vi "IRISS_FPGA_IO_RIO.vi"() -> ()   [LabVIEW 2016]
doc: "This VI contains a basic quadrature decoder which is reset asynchronously upon clicking the reset button."
uses:
  <vilib>/Platform/TimedLoop/XDataNode/timing_clust.ctl
  <vilib>/Platform/TimedLoop/XDataNode/nitl_modes.ctl
  <vilib>/Platform/TimedLoop/XDataNode/wakeup.ctl
  <vilib>/rvi/Emulation/niFpgaGetClockAttributes.vi
  <vilib>/rvi/Emulation/niFpgaSctlEmulationGetInTimedLoop.vi
  <vilib>/rvi/Emulation/niFpgaEmulationReportErrorSimple.vi
  <vilib>/rvi/eio/common/nirviEmuTemplateMethod_errors.vi
  <vilib>/rvi/Emulation/niFpgaCriticalErrorInLSC.vi
  <vilib>/eio/EIONode/EIONode.xnode
  <vilib>/platform/TimedLoop/XDataNode/XDataNode.xnode
  <vilib>/Platform/TimedLoop/XDataNode/XDNodeRunTimeDep.lvlib
  Library/KevinLibraryAll/labview/KevLib01.lvlib
panel:
  in  "Reset 9":bool
  in  "Reset 10":bool
  in  "Reset 14":bool
  in  "Period (Ticks)":u32=2000
  out "Home OCT z":bool
  in  "DIR Y":bool
  in  "INHB Y":bool
  out "FAULT Y":bool
  out "Position Y":i32
  out "JumpBy2Error Y":i16
  in  "Reset Y":bool
  in  "Y DC":fxp<+,32,0>
  in  "DIR X":bool
  in  "INHB X":bool
  out "FAULT X":bool
  out "Position X":i32
  out "JumpBy2Error X":i16
  in  "Reset X":bool
  in  "DIR Z":bool
  in  "INHB Z":bool
  out "FAULT Z":bool
  out "Position Z":i32
  out "JumpBy2Error Z":i16
  in  "Reset Z":bool
  in  "Z DC":fxp<+,32,0>
  in  "X DC":fxp<+,32,0>
  out "Home L4":bool
  out "Home L1":bool
  out "Home L2":bool
  out "Home L3":bool
  in  "Positive Direction C1-4":bool
  out "JumpBy2Error C1-4":i16
  out "32 bit Position C1-4":i32
  in  "Reset C1-4":bool
  in  "Positive Direction C1-1":bool
  out "JumpBy2Error C1-1":i16
  out "32 bit Position C1-1":i32
  in  "Reset C1-1":bool
  out "32 bit Position 17":i32
  in  "Reset 17":bool
  in  "Positive Direction 17":bool
  out "JumpBy2Error 17":i16
  out "32 bit Position 16":i32
  in  "Reset 16":bool
  in  "Positive Direction 16":bool
  out "JumpBy2Error 16":i16
  out "32 bit Position 15":i32
  in  "Reset 15":bool
  in  "Positive Direction 15":bool
  out "JumpBy2Error 15":i16
  out "32 bit Position 13":i32
  in  "Reset 13":bool
  in  "Positive Direction 13":bool
  out "JumpBy2Error 13":i16
  in  "Reset 12":bool
  in  "Reset 11":bool
  out "JumpBy2Error 3":i16
  in  "Positive Direction 3":bool
  out "JumpBy2Error 1":i16
  in  "Positive Direction 1":bool
  out "AI":i16[](array[numeric])
  out "32 bit Position 3":i32
  in  "Reset 3":bool
  in  "AO":i16[](array[numeric])=[0, 0, 0, 0, 0, 0, 0, 0]
  out "32 bit Position 1":i32
  in  "Reset 1":bool
  # "Accurus Buttons"
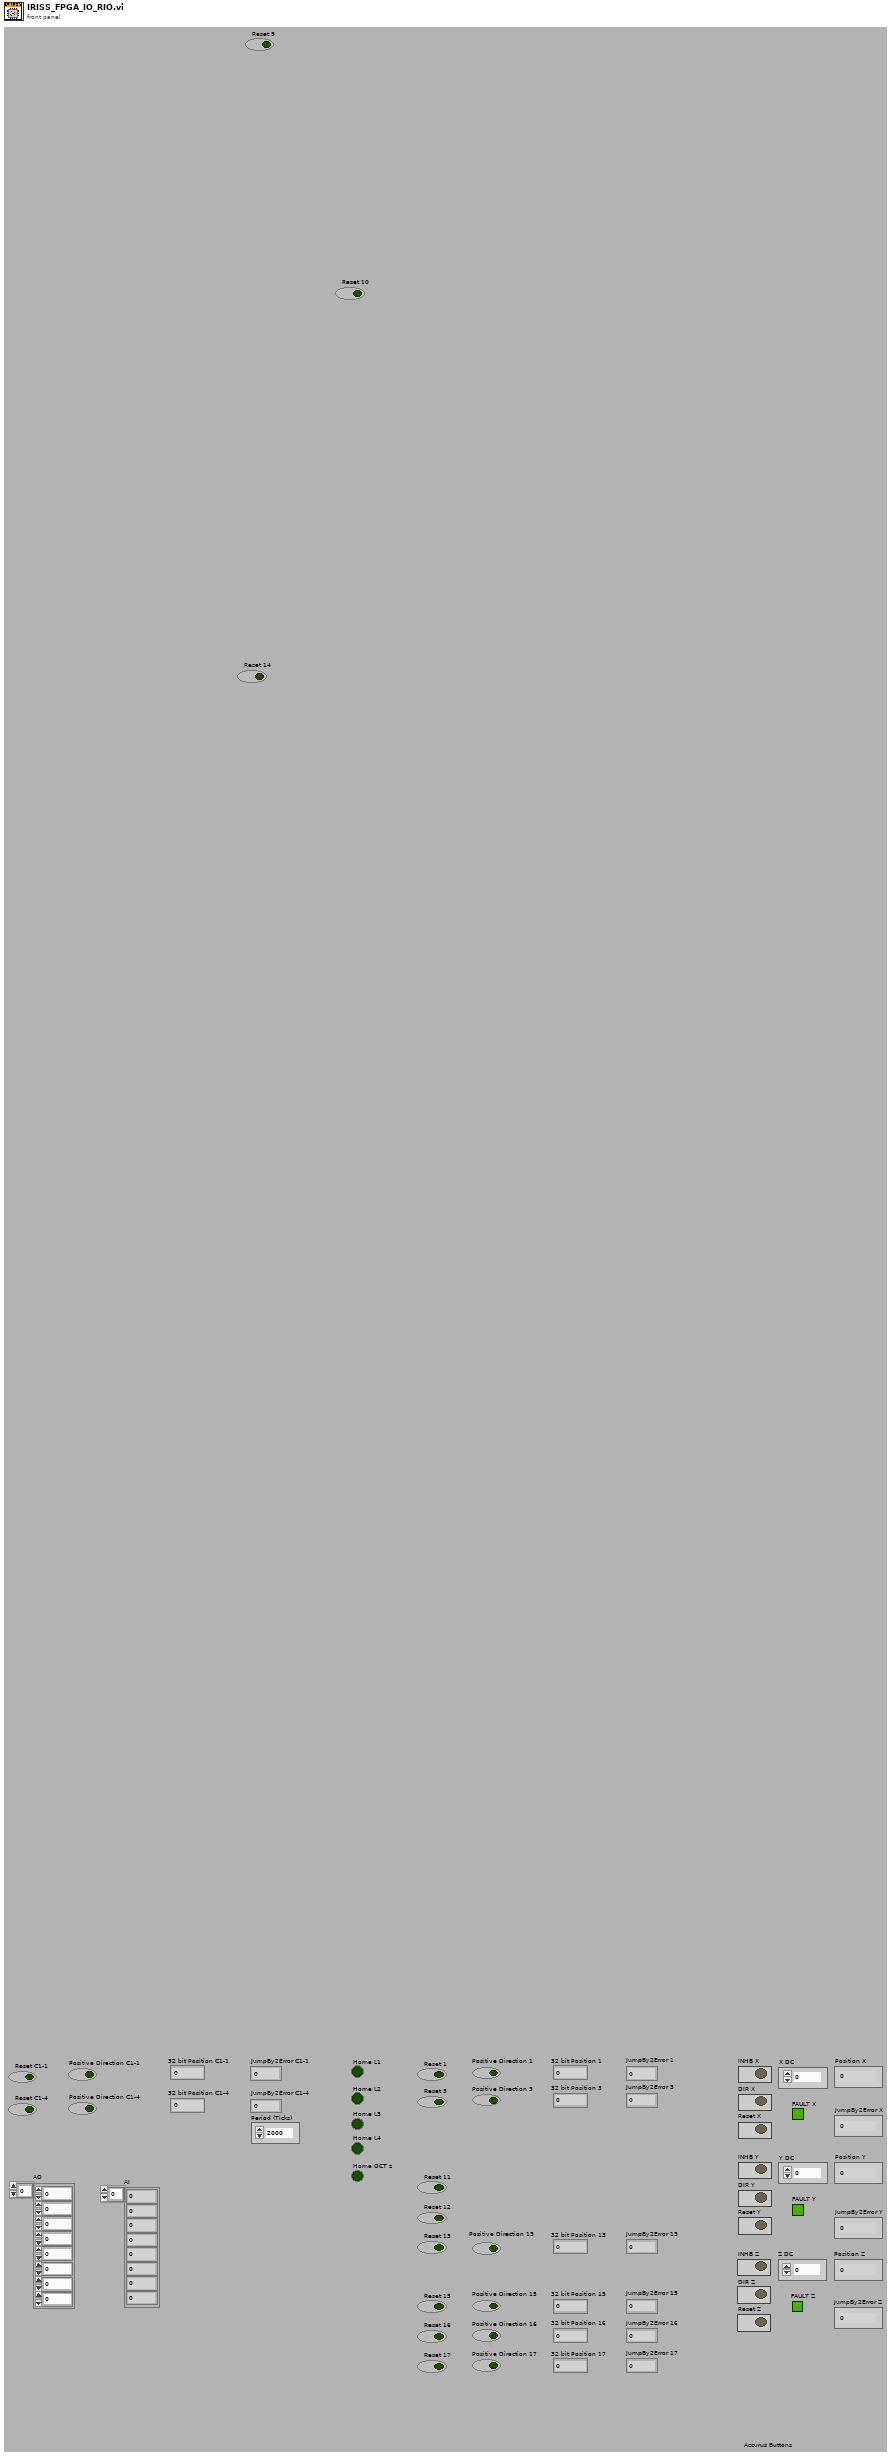
[diagram p1: front panel]
types:
  T1 = typedef "XDNodeRunTimeDep.lvlib/timing_clust.ctl" = cluster{"Expected End [f-1]":u64, "Actual End [f-1]":u64, "Finished Late? [f-1]":bool, "Expected End [i-1]":u64, "Actual End [i-1]":u64, "Finished Late? [i-1]":bool, "Expected Start [i]":u64, "Actual Start [i]":u64, "Expected Start [f]":u64, "Actual Start [f]":u64, "Source Name":string, "Structure Name":string, "Period":i64, "Deadline":i64, "Offset":i64, "Start":i64, "Priority":i32, "Timeout":i32, "Mode":T2, "Wakeup Reason":T3, "Error":errorcluster, "Source Type":string, "Secondary Source Type":string, "Global End Time":u64, "Global Start Time":u64, "Frame Duration":u64, "Iteration Duration":u64, "Assigned CPU":i32, "I/O Scan Engine Mode":u32}
  T2 = typedef "XDNodeRunTimeDep.lvlib/nitl_modes.ctl" = enum32{"No Change", "Process missed periods, maintain original phase", "Discard missed periods, maintain original phase", "Process missed periods, ignore original phase", "Discard missed periods, ignore original phase"}
  T3 = typedef "XDNodeRunTimeDep.lvlib/wakeup.ctl" = enum32{"Normal", "Aborted", "Asynchronous wakeup", "Timing source error", "Timed loop error", "Timeout"}
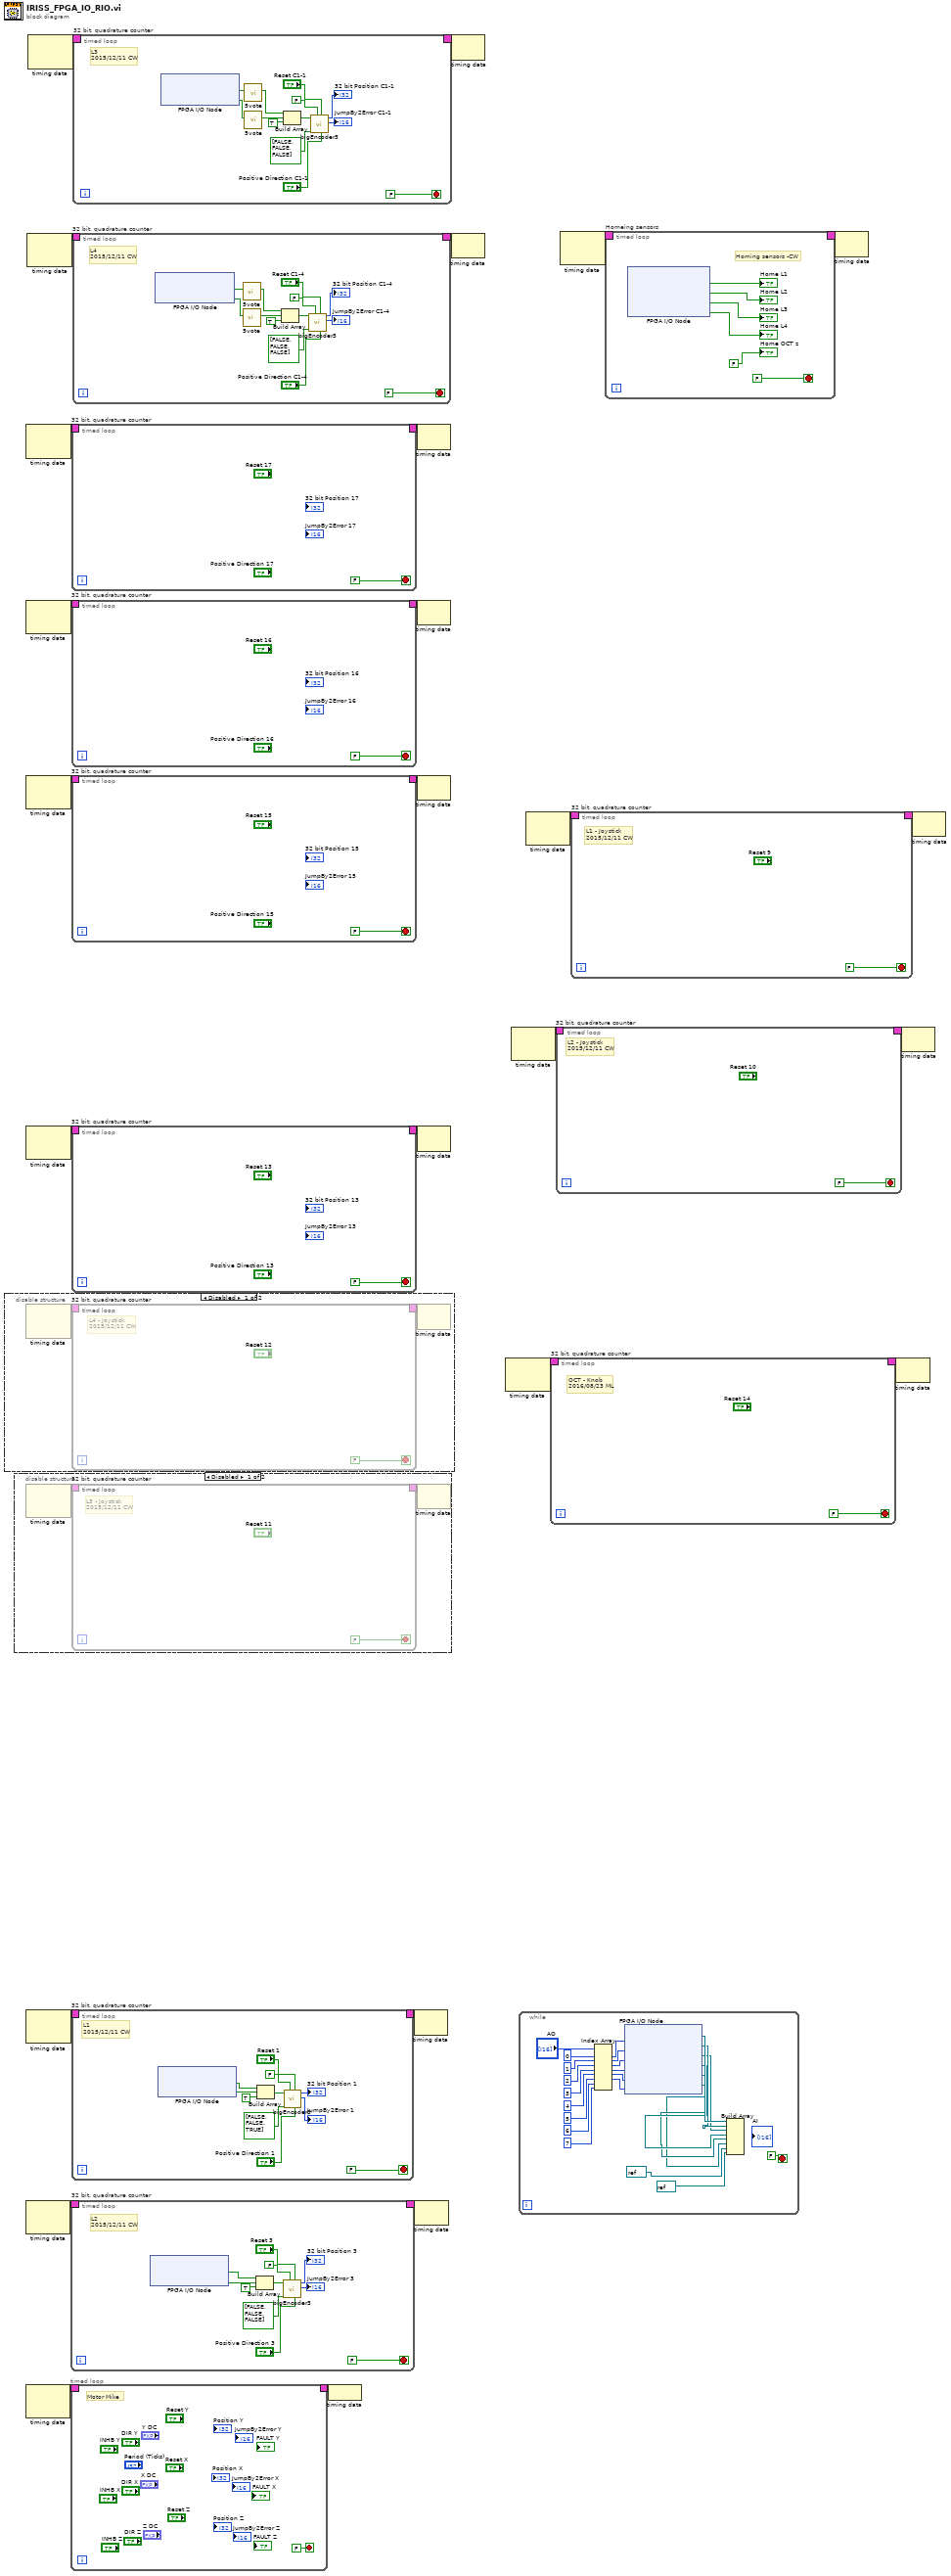
[diagram p0: block diagram]
diagram:
  n1 = disable-structure shown="Disabled" {
    frame Disabled {
      n2 = node-c288() -> (w28:T1)  [unwired: 2 out]
      n3 = timed-loop "32 bit, quadrature counter" {
        timing-out: [_] -> w27
        timing: w28 -> [_]
        stop <- FALSE stop-if-true
        # "L4 - Joystick\n2015/12/11 CW"
      }
      n4 = node-c288(w27) -> ()  [unwired: 1 out]
    }
    frame Enabled {
    }
  }
  n5 = disable-structure shown="Disabled" {
    frame Disabled {
      n6 = node-c288() -> (w35:T1)  [unwired: 2 out]
      n7 = timed-loop "32 bit, quadrature counter" {
        timing-out: [_] -> w34
        timing: w35 -> [_]
        stop <- FALSE stop-if-true
        # "L3 - Joystick\n2015/12/11 CW"
      }
      n8 = node-c288(w34) -> ()  [unwired: 1 out]
    }
    frame Enabled {
    }
  }
  n9 = node-c288() -> (w24:T1)  [unwired: 2 out]
  n10 = node-c288() -> (w8:T1)  [unwired: 2 in]
  n11 = node-c288() -> (w16:T1)  [unwired: 2 out]
  n12 = node-c288() -> (w18:T1)  [unwired: 2 out]
  n13 = node-c288() -> (w20:T1)  [unwired: 2 out]
  n14 = node-c288() -> (w22:T1)  [unwired: 2 out]
  n15 = node-c288() -> (w25:T1)  [unwired: 2 out]
  n16 = node-c288() -> (w12:T1)  [unwired: 2 out]
  n17 = node-c288() -> (w14:T1)  [unwired: 2 out]
  n18 = timed-loop "32 bit, quadrature counter" {
    timing-out: [_] -> w23
    timing: w24 -> [_]
    stop <- FALSE stop-if-true
    # "L2\n2015/12/11 CW"
    n19 = xnode "FPGA I/O Node"() -> ("ConnectorA/DIO2"=w44:bool, "ConnectorA/DIO3"=w43:bool)  [unwired: 2 in, 2 out]
    n20 = Build Array(w44, w43, TRUE ("element")) -> (w50:bool[])
    n21 = call "bigEncoder3.vi"("Positive Direction"="Positive Direction 3", "ForceReset"="Reset 3", "Allow C Reset?"=FALSE, "Reset Array"=bool[] [FALSE, FALSE, FALSE], "Encoder Array"=w50) -> ("JumpBy2Error"=→"JumpBy2Error 3":i16, "Position"=→"32 bit Position 3":i32)  [unwired: 5 out]
  }
  n22 = timed-loop {
    timing: w8 -> [_]
    timing-out: [_] -> w7
    stop <- FALSE stop-if-true
    # "Motor Mike"
  }
  n23 = timed-loop "32 bit, quadrature counter" {
    timing-out: [_] -> w15
    timing: w16 -> [_]
    stop <- FALSE stop-if-true
  }
  n24 = timed-loop "32 bit, quadrature counter" {
    timing-out: [_] -> w17
    timing: w18 -> [_]
    stop <- FALSE stop-if-true
  }
  n25 = timed-loop "32 bit, quadrature counter" {
    timing-out: [_] -> w19
    timing: w20 -> [_]
    stop <- FALSE stop-if-true
  }
  n26 = timed-loop "32 bit, quadrature counter" {
    timing-out: [_] -> w21
    timing: w22 -> [_]
    stop <- FALSE stop-if-true
  }
  n27 = timed-loop "32 bit, quadrature counter" {
    timing-out: [_] -> w26
    timing: w25 -> [_]
    stop <- FALSE stop-if-true
    # "L1\n2015/12/11 CW"
    n28 = xnode "FPGA I/O Node"() -> ("ConnectorA/DIO0"=w78:bool, "ConnectorA/DIO1"=w77:bool)  [unwired: 2 in, 2 out]
    n29 = Build Array(w78, w77, TRUE ("element")) -> (w76:bool[])
    n30 = call "bigEncoder3.vi"("Positive Direction"="Positive Direction 1", "ForceReset"="Reset 1", "Allow C Reset?"=FALSE, "Reset Array"=bool[] [FALSE, FALSE, TRUE], "Encoder Array"=w76) -> ("JumpBy2Error"=→"JumpBy2Error 1":i16, "Position"=→"32 bit Position 1":i32)  [unwired: 5 out]
  }
  n31 = timed-loop "32 bit, quadrature counter" {
    timing-out: [_] -> w11
    timing: w12 -> [_]
    stop <- FALSE stop-if-true
    # "L4\n2015/12/11 CW"
    n32 = xnode "FPGA I/O Node"() -> ("ConnectorA/DIO6"=w85:bool, "ConnectorA/DIO7"=w84:bool)  [unwired: 2 in, 2 out]
    n33 = call "5vote.vi"("Input"=w85) -> ("vote5"=w82:bool)  [unwired: 10 in]
    n34 = call "5vote.vi"("Input"=w84) -> ("vote5"=w83:bool)  [unwired: 10 in]
    n35 = Build Array(w82, w83, TRUE ("element")) -> (w93:bool[])
    n36 = call "bigEncoder3.vi"("Positive Direction"="Positive Direction C1-4", "ForceReset"="Reset C1-4", "Allow C Reset?"=FALSE, "Reset Array"=bool[] [FALSE, FALSE, FALSE], "Encoder Array"=w93) -> ("JumpBy2Error"=→"JumpBy2Error C1-4":i16, "Position"=→"32 bit Position C1-4":i32)  [unwired: 5 out]
  }
  n37 = timed-loop "32 bit, quadrature counter" {
    timing-out: [_] -> w13
    timing: w14 -> [_]
    stop <- FALSE stop-if-true
    # "L3\n2015/12/11 CW"
    n38 = xnode "FPGA I/O Node"() -> ("ConnectorA/DIO4"=w100:bool, "ConnectorA/DIO5"=w99:bool)  [unwired: 2 in, 2 out]
    n39 = call "5vote.vi"("Input"=w100) -> ("vote5"=w97:bool)  [unwired: 10 in]
    n40 = call "5vote.vi"("Input"=w99) -> ("vote5"=w98:bool)  [unwired: 10 in]
    n41 = Build Array(w97, w98, TRUE ("element")) -> (w108:bool[])
    n42 = call "bigEncoder3.vi"("Positive Direction"="Positive Direction C1-1", "ForceReset"="Reset C1-1", "Allow C Reset?"=FALSE, "Reset Array"=bool[] [FALSE, FALSE, FALSE], "Encoder Array"=w108) -> ("JumpBy2Error"=→"JumpBy2Error C1-1":i16, "Position"=→"32 bit Position C1-1":i32)  [unwired: 5 out]
  }
  n43 = node-c288(w7) -> ()
  n44 = node-c288(w26) -> ()  [unwired: 1 out]
  n45 = node-c288(w23) -> ()  [unwired: 1 out]
  n46 = node-c288(w15) -> ()  [unwired: 1 out]
  n47 = node-c288(w17) -> ()  [unwired: 1 out]
  n48 = node-c288(w19) -> ()  [unwired: 1 out]
  n49 = node-c288(w21) -> ()  [unwired: 1 out]
  n50 = node-c288(w11) -> ()  [unwired: 1 out]
  n51 = node-c288(w13) -> ()  [unwired: 1 out]
  n52 = node-c288() -> (w6:T1)  [unwired: 2 out]
  n53 = node-c288() -> (w4:T1)  [unwired: 2 out]
  n54 = while {
    stop <- FALSE stop-if-true
    n55 = Index Array(array="AO", index #1=0 ("index"), index #2=1 ("index"), index #3=2 ("index"), index #4=3 ("index"), index #5=4 ("index"), index #6=5 ("index"), index #7=6 ("index"), index #8=7 ("index")) -> (element #1=w126:i16, element #2=w125:i16, element #3=w124:i16, element #4=w123:i16, element #5=w122:i16, element #6=w121:i16)  [unwired: 2 out]
    n56 = xnode "FPGA I/O Node"("ConnectorA/AO0"=w126, "ConnectorA/AO1"=w125, "ConnectorB/AO0"=w124, "ConnectorB/AO1"=w123, "ConnectorC/AO0"=w122, "ConnectorC/AO1"=w121) -> ("FPGA I/O Out"=w119:refnum<k21>, "FPGA I/O Out"=w118:refnum<k21>, "FPGA I/O Out"=w117:refnum<k21>, "FPGA I/O Out"=w116:refnum<k21>, "FPGA I/O Out"=w115:refnum<k21>, "FPGA I/O Out"=w114:refnum<k21>)  [unwired: 6 in]
    n57 = Build Array(w119, w118, w117, w116, w115, w114, refnum<k21> refnum ("element"), refnum<k21> refnum ("element")) -> ()  [unwired: 1 out]
  }
  n58 = node-c288() -> (w2:T1)  [unwired: 2 out]
  n59 = timed-loop "32 bit, quadrature counter" {
    timing-out: [_] -> w5
    timing: w6 -> [_]
    stop <- FALSE stop-if-true
    # "OCT - Knob\n2016/08/23 ML"
  }
  n60 = timed-loop "32 bit, quadrature counter" {
    timing-out: [_] -> w3
    timing: w4 -> [_]
    stop <- FALSE stop-if-true
    # "L2 - Joystick\n2015/12/11 CW"
  }
  n61 = node-c288() -> (w10:T1)  [unwired: 2 out]
  n62 = timed-loop "32 bit, quadrature counter" {
    timing-out: [_] -> w1
    timing: w2 -> [_]
    stop <- FALSE stop-if-true
    # "L1 - Joystick\n2015/12/11 CW"
  }
  n63 = timed-loop "Homeing sensors" {
    timing-out: [_] -> w9
    timing: w10 -> [_]
    stop <- FALSE stop-if-true
    # "Homing sensors -CW"
    n64 = xnode "FPGA I/O Node"() -> ("ConnectorA/DIO8"=→"Home L1":bool, "ConnectorA/DIO9"=→"Home L2":bool, "ConnectorA/DIO10"=→"Home L3":bool, "ConnectorA/DIO11"=→"Home L4":bool)  [unwired: 4 in, 4 out]
    "Home OCT z" <- FALSE ("Home OCT z")
  }
  n65 = node-c288(w9) -> ()  [unwired: 1 out]
  n66 = node-c288(w5) -> ()  [unwired: 1 out]
  n67 = node-c288(w3) -> ()  [unwired: 1 out]
  n68 = node-c288(w1) -> ()  [unwired: 1 out]
